vi "RVC Orthogonal Rotation Matrix.vi"() -> ()   [LabVIEW 2014]
uses:
  <vilib>/Analysis/_algsub.llb/Vector Norm.vi
  <vilib>/Analysis/_algsub.llb/Real Vector Norm.vi
  <vilib>/Analysis/baseanly.llb/Outer Product.vi
  <vilib>/Analysis/baseanly.llb/Real Outer Product.vi
  <vilib>/robotics/Kinematics/Create Lie Group Matrix.vi
  <vilib>/Analysis/7linalg.llb/Create Special Matrix.vi
  <vilib>/Analysis/7linalg.llb/Create Special Real Matrix.vi
  <vilib>/Analysis/Matrix/Numeric/Multiply/Multiply.vi
  <vilib>/Analysis/Matrix/Numeric/Multiply/Multiply - RM,R.vi
  <vilib>/Analysis/Matrix/Numeric/Multiply/Multiply - R,RM.vi
  <vilib>/Analysis/Matrix/Numeric/Add/Add.vi
  <vilib>/Analysis/Matrix/Numeric/Add/Add - RM,RM.vi
  <vilib>/robotics/Kinematics/NI_Kinematics.lvlib
panel:
  in  "stop":bool
  in  "angle (degree)":dbl(slide)=1.5707963267948966 scale=0.0..360.0
  in  "Axis":u16(ring) items=["Rotate X", "Rotate Y", "Rotate Z"]
  out "3D Transformation":refnum<vi>(3d-picture)
  in  "Axis to rotate":u16(ring) items=["Rotate X", "Rotate Y", "Rotate Z"]
  in  "angle (multiple of pi)":dbl(slide)=1.5707963267948966 scale=0.0..2.0
  out "transformation matrix 2":picture
  out "3D Picture":refnum<vi>(3d-picture)
  out "transformation matrix":picture
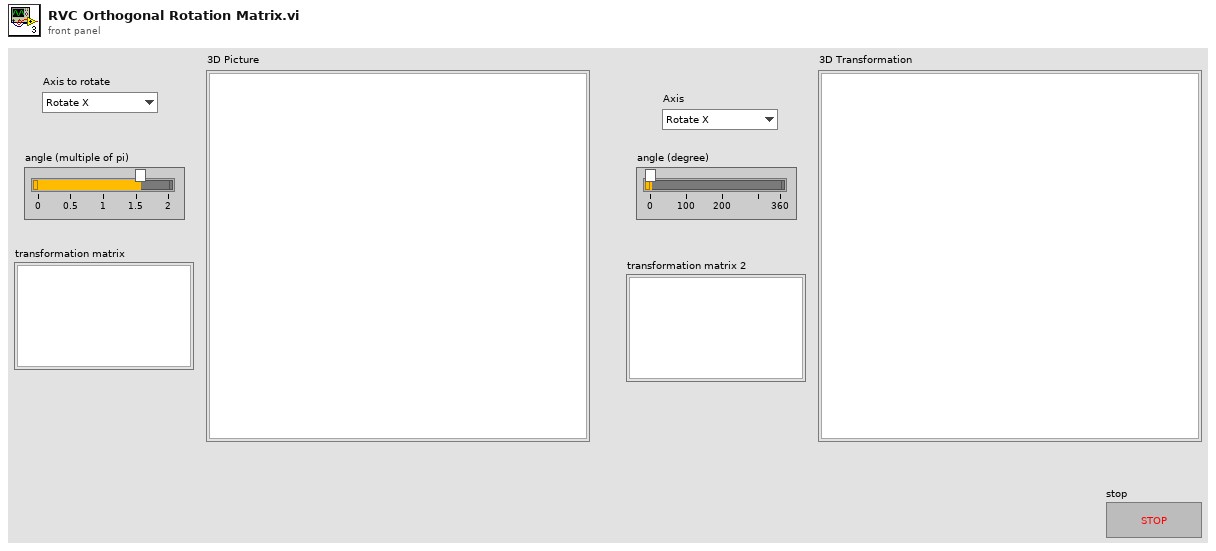
[diagram p1: front panel]
types:
  T1 = typedef "NI_Matrix.lvlib/RealMatrix.ctl" = dbl[][]
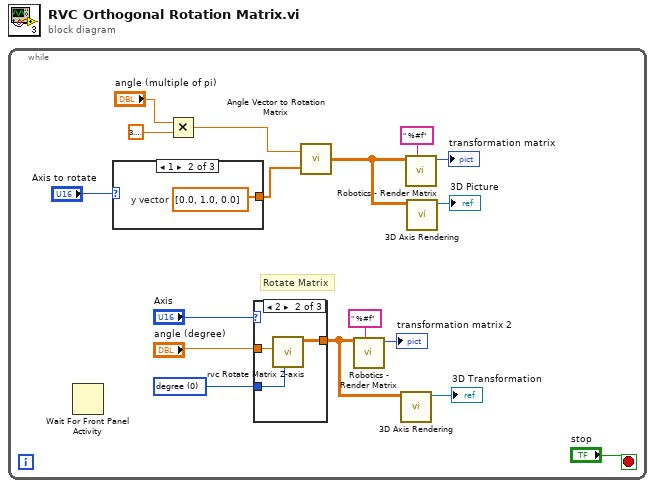
[diagram p0: block diagram]
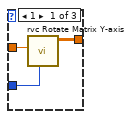
[diagram p2: hidden frame]
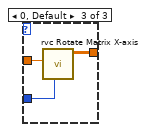
[diagram p3: hidden frame]
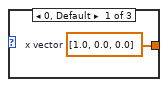
[diagram p4: hidden frame]
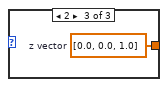
[diagram p5: hidden frame]
diagram:
  n1 = while {
    stop <- "stop" stop-if-true
    w6 = u16 0 items=["degree", "radians"] ("angle unit")
    # "Rotate Matrix"
    n2 = Wait For Front Panel Activity() -> ()  [unwired: 3 in, 1 out]
    n3 = case shown="1" "Axis to rotate" {
      tunnel: [w27 w28 w29] -> w14
      frame 0, Default {
        w27 = dbl[] [1.0, 0.0, 0.0]  # x vector
      }
      frame 1 {
        w28 = dbl[] [0.0, 1.0, 0.0]  # y vector
      }
      frame 2 {
        w29 = dbl[] [0.0, 0.0, 1.0]  # z vector
      }
    }
    n4 = Multiply(x="angle (multiple of pi)", y=3.141592653589793) -> (x*y=w2:dbl)
    n5 = case shown="2" "Axis" {
      tunnel: [w20 w23 w26] -> w12
      tunnel: "angle (degree)" -> [w19 w22 w25]
      tunnel: w6 -> [w18 w21 w24]
      frame 1 {
        n6 = call "rvc Rotate Matrix Y-axis.vi"("angle unit"=w18, "angle"=w19) -> ("rotation matrix"=w20:T1)  [unwired: 9 in]
      }
      frame 2 {
        n7 = call "rvc Rotate Matrix Z-axis.vi"("angle unit"=w21, "angle"=w22) -> ("rotation matrix"=w23:T1)  [unwired: 9 in]
      }
      frame 0, Default {
        n8 = call "rvc Rotate Matrix X-axis.vi"("angle unit"=w24, "angle"=w25) -> ("rotation matrix"=w26:T1)  [unwired: 9 in]
      }
    }
    n9 = call <vilib>:"Angle Vector to Rotation Matrix.vi"("vector"=w14, "angle"=w2) -> ("rotation matrix"=w9:T1)
    n10 = call "Robotics - Render Matrix.vi"("format string"=" %#f", "A"=w12) -> ("picture out"=→"transformation matrix 2":picture)  [unwired: 9 in]
    n11 = call "3D Axis Rendering.vi"("rotation matrix"=w12) -> ("SceneNode out"=→"3D Transformation":refnum<vi>)  [unwired: 10 in]
    n12 = call "Robotics - Render Matrix.vi"("format string"=" %#f", "A"=w9) -> ("picture out"=→"transformation matrix":picture)  [unwired: 9 in]
    n13 = call "3D Axis Rendering.vi"("rotation matrix"=w9) -> ("SceneNode out"=→"3D Picture":refnum<vi>)  [unwired: 10 in]
  }
